vi "Define Integer.vi"(7 "add ifndef/endif (F)":bool, 9 "Value":i64, 10 "Name":string, 11 "String in":string) -> (3 "String out":string)   [LabVIEW 2014, in "C Header Generator.lvlib"]
uses:
  C Header Generator.lvlib
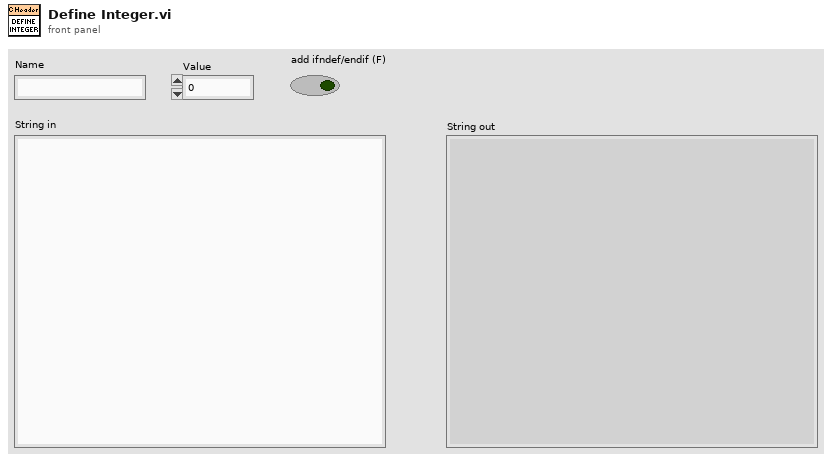
[diagram p1: front panel]
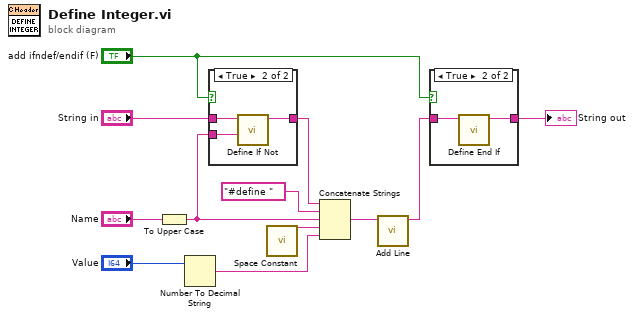
[diagram p0: block diagram]
diagram:
  n1 = To Upper Case(1:"Name") -> (0:w2:string)
  n2 = Number To Decimal String(number="Value") -> (decimal integer string=w8:string)  [unwired: 1 in]
  n3 = case shown="True" "add ifndef/endif (F)" {
    tunnel: "String in" -> [w13 w16]
    tunnel: [w13 w15] -> w5
    tunnel: w2 -> [_ w14]
    frame False {
    }
    frame True {
      n4 = call "Define If Not.vi"("token string"=w14, "String in"=w16) -> ("String out"=w15:string)  [unwired: 9 in]
    }
  }
  n5 = call <vilib>:"Space Constant.vi"() -> ("String"=w9:string)
  n6 = Concatenate Strings(w5, "#define ", w2, w9, w8) -> (w7:string)
  n7 = call "Add Line.vi"("String in"=w7) -> ("String out"=w4:string)  [unwired: 10 in]
  n8 = case shown="True" "add ifndef/endif (F)" {
    tunnel: w4 -> [w17 w19]
    tunnel: [w17 w18] -> w3
    frame False {
    }
    frame True {
      n9 = call "Define End If.vi"("String in"=w19) -> ("String out"=w18:string)  [unwired: 10 in]
    }
  }
  "String out" <- w3
